vi "Set clear and shutter.vi"(7 "# of clearing cycles":u16, 8 "error in (no error)":errorcluster, 9 "Shutter mode":T2 items=["Never", "Pre-exposure", "Pre-sequence", "Pre-trigger"], 10 "Clear mode":T1 items=["Never", "Pre-exposure", "Pre-sequence", "Post-sequence", "Pre- and post-sequence", "Pre-exp and post-seq"], 11 "camera handle in":i16) -> (0 "error out":errorcluster, 3 "camera handle out":i16)   [LabVIEW 2012]
uses:
  Shutter mode.ctl
  Clear mode.ctl
  Visual Studio/Cascade wrapper/Release/Cascade wrapper.dll
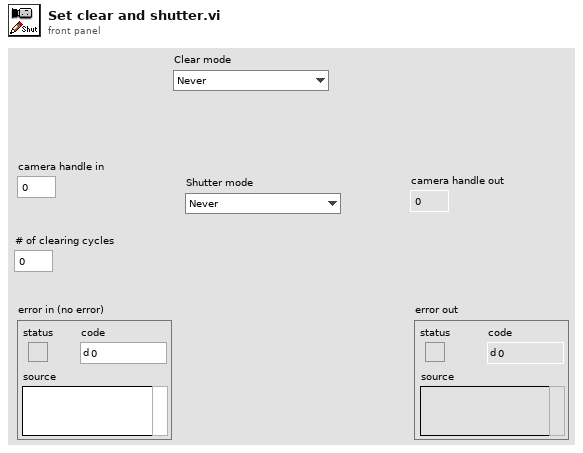
[diagram p1: front panel]
types:
  T1 = typedef "Clear mode.ctl" = i32
  T2 = typedef "Shutter mode.ctl" = i32
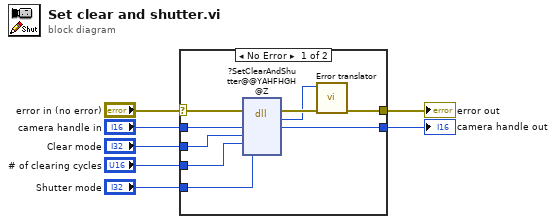
[diagram p0: block diagram]
diagram:
  n1 = case shown="No Error" "error in (no error)" {
    selector: "error in (no error)" -> [w16 w18]
    tunnel: "camera handle in" -> [w15 w17]
    tunnel: "Clear mode" -> [w14 _]
    tunnel: "# of clearing cycles" -> [w13 _]
    tunnel: "Shutter mode" -> [w12 _]
    tunnel: [w9 w18] -> w2
    tunnel: [w8 w17] -> w1
    frame No Error {
      n2 = dll-call lib="C:/moroder/Cascade wrapper/Visual Studio/Cascade wrapper/Release/Cascade wrapper.dll" fn="?SetClearAndShutter@@YAHFHGH@Z"(error in=w16, "camera handle"=w15, "clear mode"=w14, "clear cycles"=w13, "shutter mode"=w12) -> (error out=w11:errorcluster, "error"=w10:i32, "camera handle"=w8:i16)  [unwired: 5 in, 1 out]
      n3 = call "Error translator.vi"("error in (no error)"=w11, "error code"=w10) -> ("error out"=w9:errorcluster)  [unwired: 9 in]
    }
    frame Error {
    }
  }
  "error out" <- w2
  "camera handle out" <- w1
